vi "Read ID.vi"(8 "error in (no error)":errorcluster, 11 "TY720 in":refnum<class "TY720.lvclass">) -> (0 "error out":errorcluster, 3 "TY720 out":refnum<class "TY720.lvclass">)   [LabVIEW 2015, in "TY720.lvclass"]
doc: "VI used to Read Hardware ID"
uses:
  TY720.lvclass
  <vilib>/Instr/_visa.llb/VISA Configure Serial Port (Instr).vi
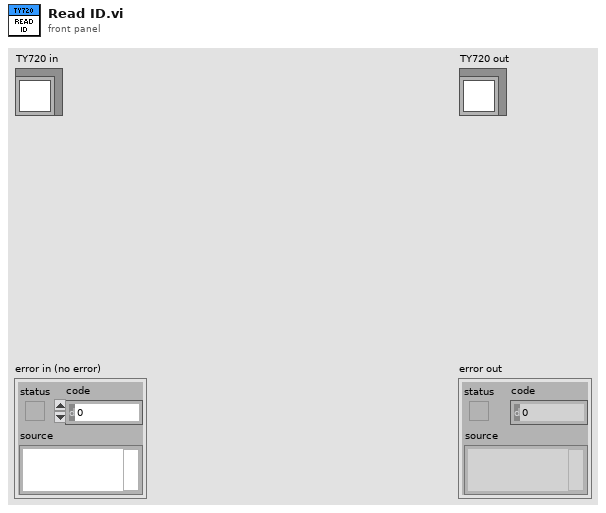
[diagram p1: front panel]
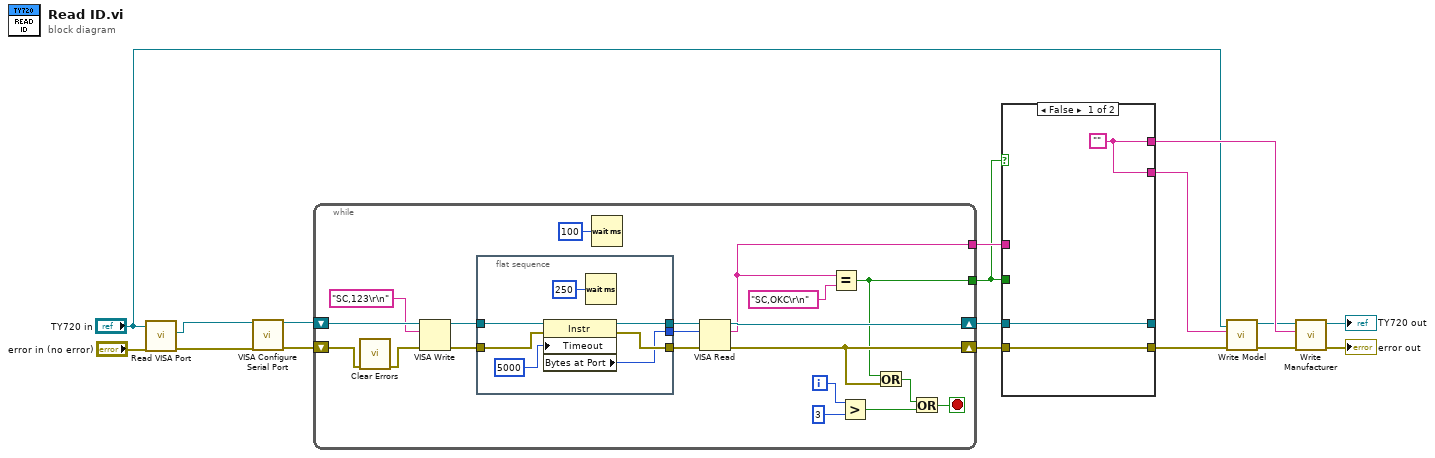
[diagram p0: block diagram]
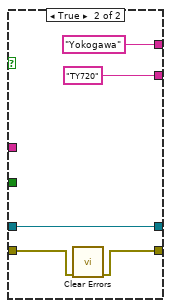
[diagram p2: hidden frame]
diagram:
  n1 = call-dynamic "Read VISA Port.vi"("error in (no error)"="error in (no error)", "Device in"="TY720 in") -> ("error out"=w3:errorcluster, "VISA Port"=w1:refnum<visa-resource-name>)  [unwired: 7 in, 1 out]
  n2 = call-poly "VISA Configure Serial Port"("VISA resource name"=w1, "error in (no error)"=w3) -> ("VISA resource name out"=w2:refnum<visa-resource-name>, "error out"=w17:errorcluster)  [unwired: 12 in]
  n3 = while {
    shift-right: [w22] -> w14
    shift-left: w17 -> [w28]
    shift-right: [w36] -> w15
    shift-left: w2 -> [w37]
    tunnel: [w19] -> w16
    tunnel: [w18] -> w13
    i -> [w30]
    stop <- w23 stop-if-true
    n4 = call <vilib>:"Clear Errors.vi"("error in (no error)"=w28) -> ("error out"=w27:errorcluster)  [unwired: 5 in, 1 out]
    n5 = VISA Write(VISA resource name=w37, write buffer="SC,123\r\n", error in (no error)=w27) -> (VISA resource name out=w34:refnum<visa-resource-name>, error out=w32:errorcluster)  [unwired: 1 out]
    n6 = flat-sequence {
      tunnel: w34 -> [w44]
      tunnel: [w42] -> w33
      tunnel: w32 -> [w41]
      tunnel: [w40] -> w31
      tunnel: [w39] -> w20
      frame #0 {
        n7 = property class="Instr"(reference=w44, error in=w41, "Timeout"=u32 5000 ("General Settings:Timeout Value")) -> (reference out=w42:refnum<visa-resource-name>, error out=w40:errorcluster, "Bytes at Port"=w39:u32)
        n8 = Wait (ms)(milliseconds to wait=u32 250) -> ()  [unwired: 1 out]
      }
    }
    n9 = Wait (ms)(milliseconds to wait=u32 100) -> ()  [unwired: 1 out]
    n10 = VISA Read(VISA resource name=w33, byte count=w20, error in (no error)=w31) -> (VISA resource name out=w36:refnum<visa-resource-name>, read buffer=w19:string, error out=w22:errorcluster)  [unwired: 1 out]
    n11 = Equal?(x=w19, y="SC,OKC\r\n") -> (x = y?=w18:bool)
    n12 = Greater?(x=w30, y=3) -> (0:w24:bool)
    n13 = Or(x=w18, y=w22) -> (x .or. y?=w21:bool)
    n14 = Or(x=w21, y=w24) -> (x .or. y?=w23:bool)
  }
  n15 = case shown="False" w13 {
    tunnel: [w47 "Yokogawa"] -> w9
    tunnel: [w47 "TY720"] -> w10
    tunnel: w16 -> [_ _]
    tunnel: [w46 w50] -> _
    tunnel: w15 -> [w46 w50]
    tunnel: [w45 w48] -> w11
    tunnel: w14 -> [w45 w49]
    tunnel: w13 -> [_ _]
    frame False {
      w47 = ""
    }
    frame True {
      n16 = call <vilib>:"Clear Errors.vi"("error in (no error)"=w49) -> ("error out"=w48:errorcluster)  [unwired: 5 in, 1 out]
    }
  }
  n17 = call-dynamic "Write Model.vi"("error in (no error)"=w11, "Model"=w10, "Device in"="TY720 in") -> ("error out"=w8:errorcluster, "Device out"=w7:refnum<class "TY720.lvclass">)  [unwired: 7 in]
  n18 = call-dynamic "Write Manufacturer.vi"("error in (no error)"=w8, "Manufacturer"=w9, "Device in"=w7) -> ("error out"=→"error out":errorcluster, "Device out"=→"TY720 out":refnum<class "TY720.lvclass">)  [unwired: 7 in]
